vi "FTW-XML-Element-GetFirstChild.vi"(0 "Element Node":refnum<k20>, 11 "error in":errorcluster) -> (4 "Element Node out":refnum<k20>, 6 "First Child Element Node":refnum<k20>, 8 "Found?":bool, 15 "error out":errorcluster)   [LabVIEW 2014]
uses:
  <resource>/objmgr/DOMUserDefRef.rc
panel:
  # "Inputs"
  # "Outputs"
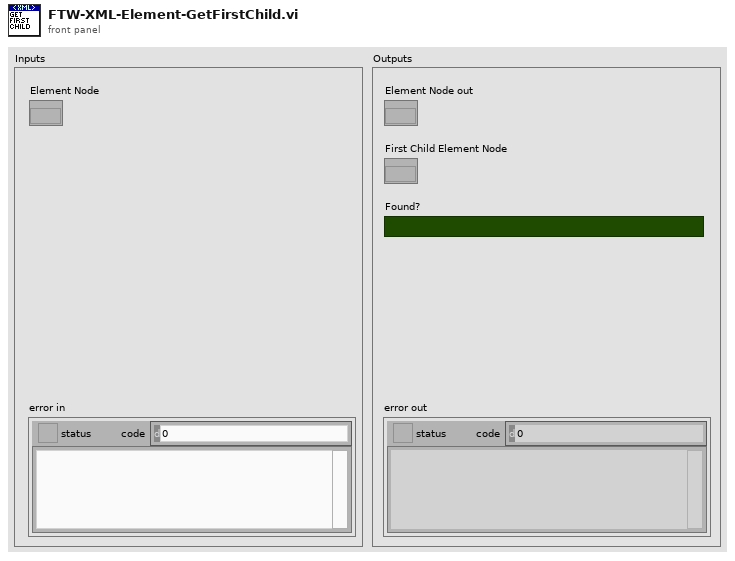
[diagram p1: front panel]
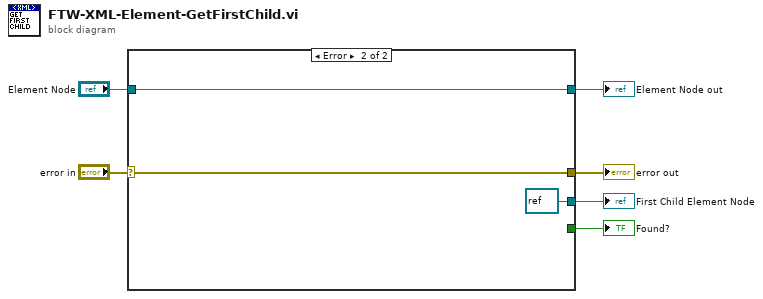
[diagram p0: block diagram]
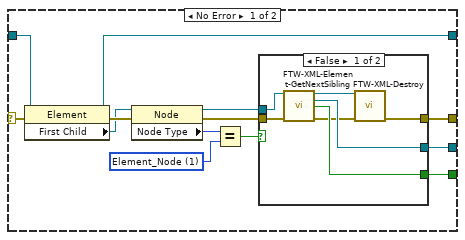
[diagram p2: hidden frame]
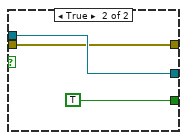
[diagram p3: hidden frame]
diagram:
  n1 = case shown="Error" "error in" {
    selector: "error in" -> [w17 w32]
    tunnel: [w13 w32] -> w6
    tunnel: "Element Node" -> [w19 w31]
    tunnel: [w18 w31] -> w3
    tunnel: [w14 refnum<k20> refnum ("FirstChild")] -> w2
    tunnel: [w12 _] -> w1
    frame No Error {
      w11 = 1 items=["Element_Node"=1, "Attribute_Node"=2, "Text_Node"=3, "CDATASection_Node"=4, "EntityReference_Node"=5, "Entity_Node"=6, "ProcessingInstruction_Node"=7, "Comment_Node"=8, "Document_Node"=9, "DocumentType_Node"=10, "DocumentFragment_Node"=11, "Notation_Node"=12] ("Node Type")
      n2 = property class="Element"(reference=w19, error in=w17) -> (reference out=w18:refnum<k20>, error out=w16:errorcluster, "First Child"=w15:refnum<k20>)
      n3 = property class="Node"(reference=w15, error in=w16) -> (reference out=w8:refnum<k20>, error out=w9:errorcluster, "Node Type"=w10:i32)
      n4 = Equal?(x=w10, y=w11) -> (x = y?=w7:bool)
      n5 = case shown="False" w7 {
        tunnel: w9 -> [w26 w28]
        tunnel: w8 -> [w25 w29]
        tunnel: [w24 w29] -> w14
        tunnel: [w23 TRUE ("Found?")] -> w12
        tunnel: [w20 w28] -> w13
        frame False {
          n6 = call "FTW-XML-Element-GetNextSibling.vi"("XML Node"=w25, "error in"=w26) -> ("XML Node out"=w22:refnum<k20>, "Next Sibling"=w24:refnum<k20>, "Found?"=w23:bool, "error out"=w21:errorcluster)  [unwired: 10 in]
          n7 = call "FTW-XML-Destroy.vi"("XML Node"=w22, "error in"=w21) -> ("error out"=w20:errorcluster)  [unwired: 13 in]
        }
        frame True {
        }
      }
    }
    frame Error {
    }
  }
  "error out" <- w6
  "Element Node out" <- w3
  "Found?" <- w1
  "First Child Element Node" <- w2
